vi "PreviewPicture.vi"(9 "Title":string, 11 "2D Picture":picture) -> ()   [LabVIEW 2015, in "Configuration Tool.lvlib"]
uses:
  Configuration Tool.lvlib
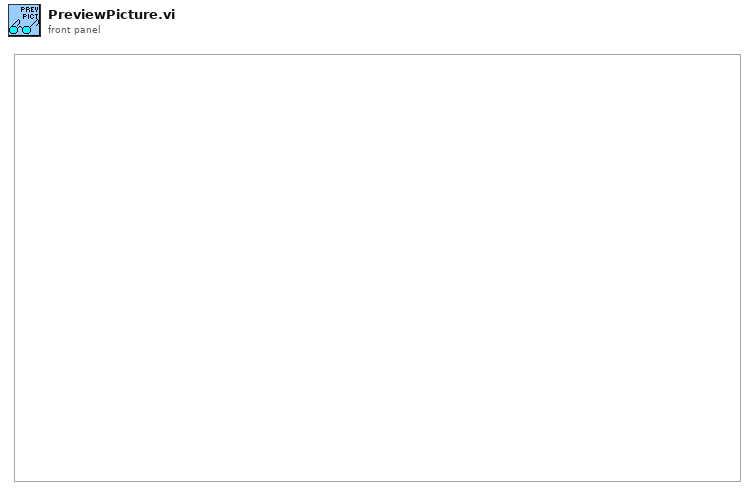
[diagram p1: front panel]
types:
  T1 = typedef "imagedata.ctl" = cluster{"image type":i32, "image depth":i32, "image":u8[], "mask":u8[], "colors":u32[], "Rectangle":cluster{"left":i16, "top":i16, "right":i16, "bottom":i16}}
  T2 = typedef "LVRectTypeDef.ctl" = cluster{"Left":i16, "Top":i16, "Right":i16, "Bottom":i16}
  T3 = cluster{"left":i16, "top":i16, "right":i16, "bottom":i16}
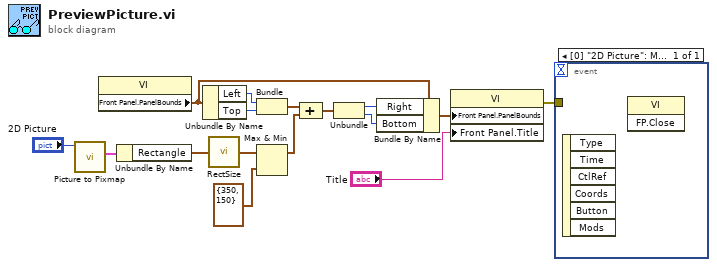
[diagram p0: block diagram]
diagram:
  n1 = call <vilib>:"Picture to Pixmap.vi"("picture"="2D Picture") -> ("image data"=w15:T1)  [unwired: 9 in, 1 out]
  n2 = property class="VI"() -> ("Front Panel.PanelBounds"=w13:T2)  [unwired: 2 in, 2 out]
  n3 = Unbundle By Name(w15) -> ("Rectangle"=w14:T3)
  n4 = Unbundle By Name(w13) -> ("Left"=w8:i16, "Top"=w9:i16)
  n5 = call <vilib>:"RectSize.vi"("rect"=w14) -> ("point"=w11:cluster{"x":i16, "y":i16})
  n6 = Bundle("Left"=w8, "Top"=w9) -> (w7:cluster{"Left":i16, "Top":i16})  [unwired: 1 in]
  n7 = Max & Min(x=w11, y=cluster{"x":i16, "y":i16} {"x"=350, "y"=150}) -> (max(x,y)=w2:cluster{"x":i16, "y":i16})  [unwired: 1 out]
  n8 = Compound Arithmetic op=ADD(w7, w2) -> (w6:cluster{i16, i16})
  n9 = Unbundle(w6) -> (w5:i16, w4:i16)
  n10 = Bundle By Name(cluster=w13, "Right"=w5, "Bottom"=w4) -> (w12:T2)
  n11 = property class="VI"("Front Panel.PanelBounds"=w12, "Front Panel.Title"="Title") -> (error out=w3:errorcluster)  [unwired: 2 in, 1 out]
  n12 = event shown="[0] \"2D Picture\": Mouse Down" {
    selector: _ -> [_]
    dyn-events: _ -> [_]
    timeout: _ -> [_]
    tunnel: w3 -> [_]
    event "2D Picture": Mouse Down {
      n13 = event-data() -> ()  [unwired: 1 in, 6 out]
      n14 = invoke class="VI" method="FP.Close"() -> ()  [unwired: 3 in, 3 out]
    }
  }
